vi "Example Custom LVClass Serialization.vi"() -> ()   [LabVIEW 2017]
uses:
  Demo LVClass Serializer.lvclass
  C:/Git/JSONtext/LVClass Serializer/JSONtext LVClass Serializer.lvclass
  <vilib>/drjdpowell/Messenging/Core Messages/Message/MSG.lvclass/MSG.ctl
  <vilib>/drjdpowell/Messenging/Core Messages/ObjectMessage/ObjectMSG.lvclass/ObjectMSG.ctl
  <vilib>/drjdpowell/Messenging/Core Messages/MSG Library/Write Message (Object).vi
  912a6c23-4bb1-4c3c-9308-e383c675d733.vi
  e1d0a090-eb0b-4084-98ba-e2f06df06374.vi
  <vilib>/drjdpowell/Messenging/Core Messages/Message/Overwrite Reply Address.vi
  <vilib>/drjdpowell/Messenging/Core Messages/ObjectMessage/Write ObjectMSG.vi
  <vilib>/drjdpowell/Messenging/Core Messages/Message/Label Message.vi
  <vilib>/drjdpowell/Messenging/Core Messages/ObjectMessage/ObjectMSG.lvclass
  C:/Program Files (x86)/National Instruments/LabVIEW 2017/vi.lib/drjdpowell/Messenging/Core Messages/Message/MSG.lvclass
  Variant to JSON Text.vi
  JSON text to Variant.vi
  <vilib>/drjdpowell/Messenging/Core Messengers/Send/Send.lvclass
  <vilib>/drjdpowell/Messenging/Core Messages/MSG Library/SendMSG.lvlib
  <vilib>/drjdpowell/Messenging/Core Messages/Message/MSG.lvclass
panel:
  out "x = y?":bool
  out "error out":errorcluster
  out "<JSON>":string
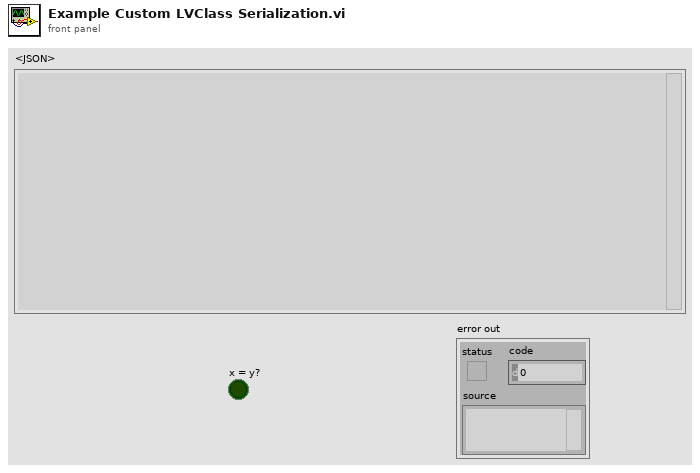
[diagram p1: front panel]
types:
  T1 = cluster{"Message":refnum<class>, "Obj":refnum<class>}
  T2 = cluster{"Message":refnum<class "MSG.lvclass">, "Obj":refnum<class "Demo LVClass Serializer.lvclass">}
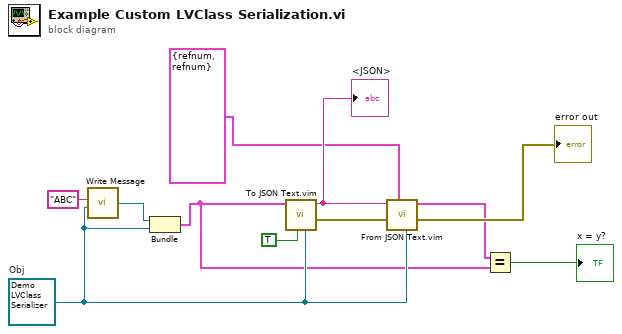
[diagram p0: block diagram]
diagram:
  w5 = refnum<class "Demo LVClass Serializer.lvclass"> refnum  # Obj
  n1 = call-poly <vilib>:"Write Message.vi"("Label"="ABC", "Contents"=w5) -> ("Message"=w4:refnum<class "MSG.lvclass">)  [unwired: 6 in]
  n2 = Bundle("Message"=w4, "Obj"=w5) -> (w3:T2)  [unwired: 1 in]
  n3 = call "To JSON Text.vim"("LVClass Serializer"=w5, "Pretty Print?"=TRUE, "Anything"=w3) -> ("error out"=w8:errorcluster, "<JSON>"=w9:string)  [unwired: 7 in]
  "<JSON>" <- w9
  n4 = call "From JSON Text.vim"("LVClass Serializer"=w5, "Data Type and Default Value"=T1 {"Message"=refnum, "Obj"=refnum} ("output cluster"), "error in (no error)"=w8, "JSON"=w9) -> ("error out"=→"error out":errorcluster, "Data out"=w1:T1)  [unwired: 6 in]
  n5 = Equal?(x=w1, y=w3) -> (x = y?=→"x = y?":bool)
